vi "Q -- range -- gate  - AND.vi"(3 "state two":T2=enum."above", 4 "state one":T2=enum."above") -> (0 "selector":T1)   [LabVIEW 2010]
uses:
  comparison control.ctl
  comparison control - double.ctl
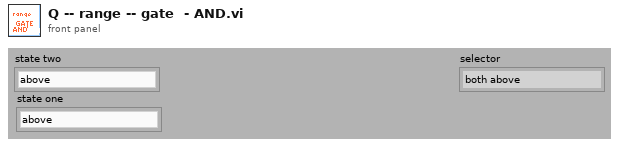
[diagram p1: front panel]
types:
  T1 = typedef "comparison control - double.ctl" = enum16{"both above", "both below", "both in range", "above , below", "below, above", "other"}
  T2 = typedef "comparison control.ctl" = enum16{"not a number", "above", "in range", "below"}
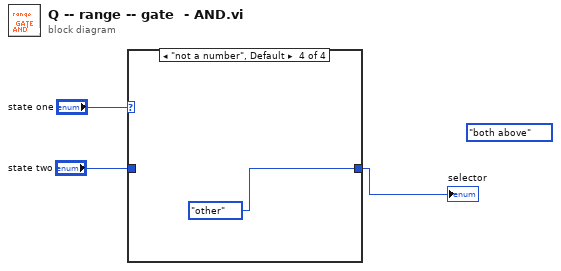
[diagram p0: block diagram]
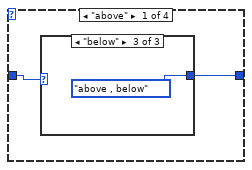
[diagram p2: hidden frame]
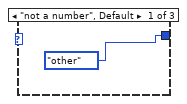
[diagram p3: hidden frame]
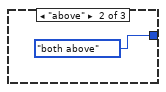
[diagram p4: hidden frame]
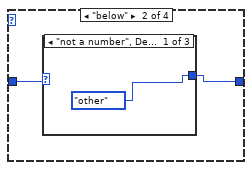
[diagram p5: hidden frame]
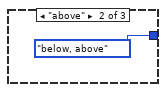
[diagram p6: hidden frame]
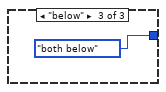
[diagram p7: hidden frame]
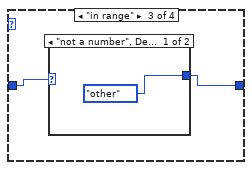
[diagram p8: hidden frame]
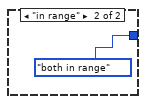
[diagram p9: hidden frame]
diagram:
  (unwired) comparison_control_-_double."both above" ("selector")
  n1 = case shown="\"not a number\", Default" "state one" {
    tunnel: [w4 w9 w15 comparison_control_-_double."other" ("selector")] -> w1
    tunnel: "state two" -> [w5 w10 w14 _]
    frame "above" {
      n2 = case shown="\"below\"" w5 {
        tunnel: [comparison_control_-_double."other" ("selector") comparison_control_-_double."both above" ("selector") comparison_control_-_double."above , below" ("selector")] -> w4
        frame "not a number", Default {
        }
        frame "above" {
        }
        frame "below" {
        }
      }
    }
    frame "below" {
      n3 = case shown="\"not a number\", Default" w10 {
        tunnel: [comparison_control_-_double."other" ("selector") comparison_control_-_double."below, above" ("selector") comparison_control_-_double."both below" ("selector")] -> w9
        frame "not a number", Default {
        }
        frame "above" {
        }
        frame "below" {
        }
      }
    }
    frame "in range" {
      n4 = case shown="\"not a number\", Default" w14 {
        tunnel: [comparison_control_-_double."other" ("selector") comparison_control_-_double."both in range" ("selector")] -> w15
        frame "not a number", Default {
        }
        frame "in range" {
        }
      }
    }
    frame "not a number", Default {
    }
  }
  "selector" <- w1
